vi "Format ITX Graph.vi"() -> ()   [LabVIEW 2019, in "ITX Commands.lvclass"]
uses:
  ITX Commands.lvclass
  typedefs/grid--enum.ctl
  typedefs/textbox_anchorcolumn--enum.ctl
  typedefs/textbox_anchorrow--enum.ctl
  typedefs/log--enum.ctl
panel:
  in  "graph/image":bool
  in  "Axes Thickness":T1
  in  "Prescale Exponent\n(0 => no change)":T1
  in  "Log Scale?":cluster{"bottom axis":T2, "left axis":T2}
  in  "Colorscale":u32[](array[colorbox])=[16711680, 16744448, 16776960, 65280, 255, 8388863, 16711935]
  in  "Textbox":T5
  in  "Grid":T6
  in  "Graph Width\n(points)":dbl
  in  "Graph Height\n(points)":dbl
  in  "Mirror? [T}":bool=TRUE
  in  "Label":T7
  in  "Wavename(s)":string[](array[string])
  # "Graph Properties"
  # "List of Commands:\nAppendtoGraph (one or more waves)\nAppendImage (one wave)\nLabel (label axes)\nModifyGraph axThick (axes thickness)\nModifyGraph grid (grid lines on graph)\nModifyGraph height (height of graph)\nModifyGraph log (log scale)\nModifyGraph mirror (mirror graph)\nModifyGraph prescaleExp (prescale exp of axes)\nModifyGraph rgb (colorscale)\nModifyGraph width (width of graph)\nTextbox"
  # "Axes Properties"
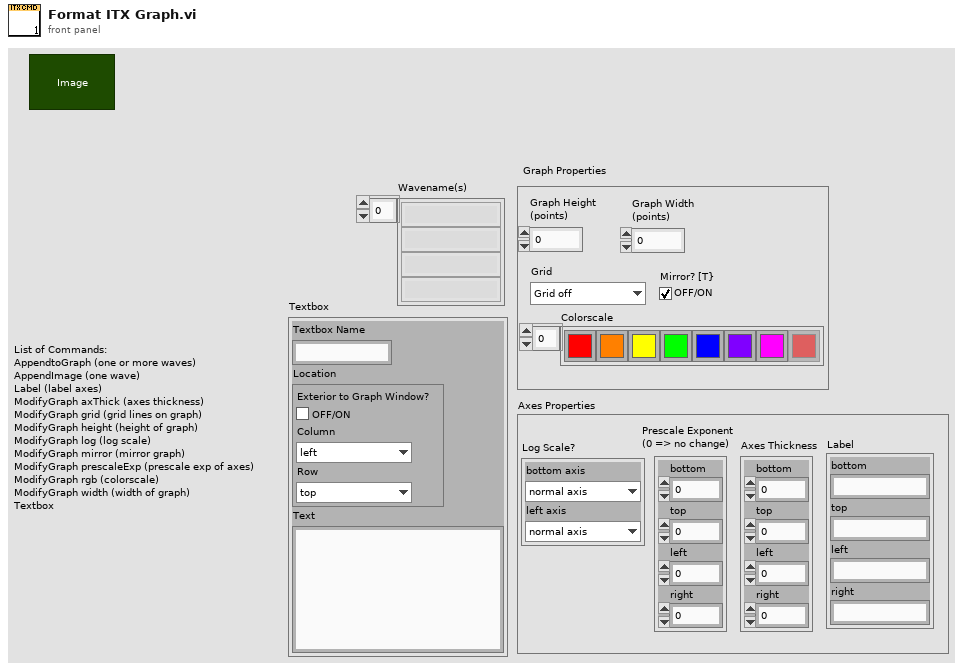
[diagram p1: front panel]
types:
  T1 = cluster{"bottom":dbl, "top":dbl, "left":dbl, "right":dbl}
  T2 = typedef "ITX Commands.lvclass/log--enum.ctl" = enum16{"normal axis", "log base 10", "log base 2"}
  T3 = typedef "ITX Commands.lvclass/textbox_anchorcolumn--enum.ctl" = enum16{"left", "middle", "right"}
  T4 = typedef "ITX Commands.lvclass/textbox_anchorrow--enum.ctl" = enum16{"top", "center", "bottom"}
  T5 = cluster{"Textbox Name":string, "Location":cluster{"Exterior to Graph Window?":bool, "Column":T3, "Row":T4}, "Text":string}
  T6 = typedef "ITX Commands.lvclass/grid--enum.ctl" = enum16{"Grid off", "Grid on", "Grid on major ticks only"}
  T7 = cluster{"bottom":string, "top":string, "left":string, "right":string}
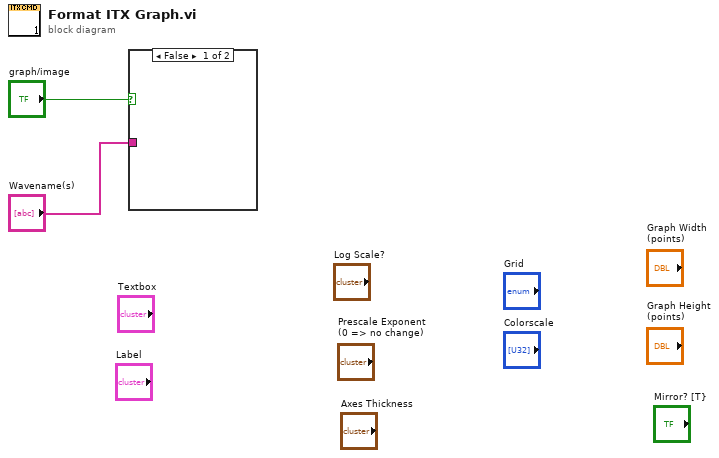
[diagram p0: block diagram]
diagram:
  n1 = case shown="False" "graph/image" {
    tunnel: "Wavename(s)" -> [_ _]
    frame False {
    }
    frame True {
    }
  }
